vi "CfgManager.Text Partial Found Test Launcher.vi"() -> ()   [LabVIEW 2013]
uses:
  <vilib>/LabVIEW Open Source Project/Unicity/Delimiter/Delimiters List.ctl
  Manager.Text/ConfigManager.Text.lvclass
  Manager.Text/ConfigManager.Text.lvclass/ConfigManager.Text.ctl
  <vilib>/LabVIEW Open Source Project/Unicity/Delimiter/Delimiter.lvclass
  Manager/ConfigManager.lvclass
panel:
  out "any found?":bool
  out "all found? 2":bool
  out "default pump config":variant
  in  "default config":path
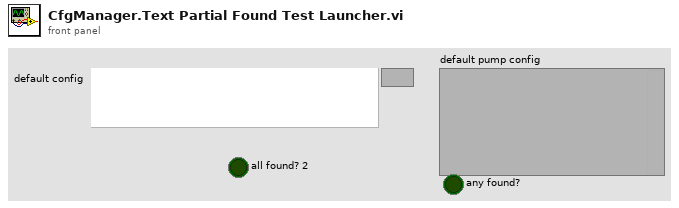
[diagram p1: front panel]
types:
  T1 = cluster{"String":string, "Numeric":dbl, "Boolean":bool}
  T2 = typedef "Delimiter.lvclass/Delimiters List.ctl" = enum16{"Default", "dot (.)", "colon (:)", "double-colon (::)", "semi-colon (;)", "underscore (_)", "double underscore (__)", "dash (-)", "double dash (--)", "backslash (\\)", "vertical bar (|)", "forward slash (/)", "chevron (>)", "double-chevron (>>)", "arrow (->)", "comma (,)", "arobas (@)", "ampersand (&)", "other"}
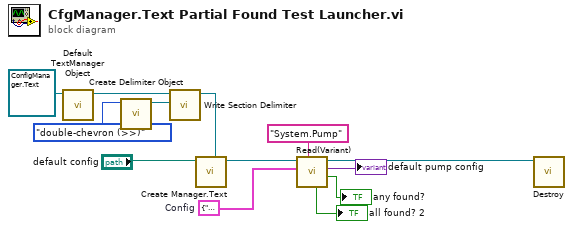
[diagram p0: block diagram]
diagram:
  w4 = T1 {"String"="", "Numeric"=0.0, "Boolean"=FALSE}  # Config
  n1 = call-dynamic "Default TextManager Object.vi"("CfgManager.Text in"=refnum<class "ConfigManager.Text.lvclass"> refnum) -> ("CfgManager.Text out"=w10:refnum<class "ConfigManager.Text.lvclass">)  [unwired: 10 in]
  n2 = call <vilib>:"Create Delimiter Object.vi"("Delimiter"=Delimiters_List."double-chevron (>>)") -> ("Delimiter"=w11:refnum<class "Delimiter.lvclass">)  [unwired: 10 in]
  n3 = call "Write Section Delimiter.vi"("Section Delimiter"=w11, "ConfigManager.Text in"=w10) -> ("ConfigManager.Text out"=w9:refnum<class "ConfigManager.Text.lvclass">)  [unwired: 9 in]
  n4 = call "Create Manager.Text.vi"("ConfigManager.Text"=w9, "filepath"="default config") -> ("ConfigManager.Text out"=w7:refnum<class "ConfigManager.Text.lvclass">)  [unwired: 7 in, 2 out]
  n5 = call "Read(Variant).vi"("Qualified Name"="System.Pump", "Type"=w4, "ConfigManager in"=w7) -> ("any found?"=→"any found?":bool, "value"=→"default pump config":variant, "ConfigManager out"=w2:refnum<class "ConfigManager.Text.lvclass">, "all found?"=→"all found? 2":bool)  [unwired: 4 in, 1 out]
  n6 = call-dynamic "Destroy.vi"("ConfigManager.Text in"=w2) -> ()  [unwired: 9 in, 2 out]
